vi "Wait for Pulse Acquired.vi"(8 "error in (no error)":errorcluster, 11 "Pulse Recorder Actor in":refnum<class "Pulse Recorder Actor.lvclass">) -> (0 "error out":errorcluster, 3 "Pulse Recorder Actor out":refnum<class "Pulse Recorder Actor.lvclass">)   [LabVIEW 2021, in "Pulse Recorder Actor.lvclass"]
uses:
  Pulse Recorder Actor.lvclass
  C:/GitHub/LabActor/Template Module/Template Module.lvclass
  C:/Program Files/National Instruments/LabVIEW 2021/vi.lib/ActorFramework/Actor/Actor.lvclass
  C:/GitHub/LabActor/Worker/Worker Actor/Worker Actor.lvclass
  Template Module/Template Module.lvclass/Template Module.ctl
  <vilib>/ActorFramework/Actor/Actor.lvclass/Actor.ctl
  Publish-Subscribe/Interfaces/Subscriber Messages/Information Msg/Information Msg.lvclass/Information Msg.ctl
  <vilib>/ActorFramework/Message Enqueuer/Message Enqueuer.lvclass/Message Enqueuer.ctl
  Pulse Recorder Actor.lvclass/Pulse Recorder Actor.ctl
  Interfaces/Pulse Recorder Messages/Wait for Pulse Acquired Msg/Wait for Pulse Acquired Msg.lvclass
  C:/Program Files/National Instruments/LabVIEW 2021/vi.lib/ActorFramework/Message/Message.lvclass
  Worker/Worker Actor/Worker Actor.lvclass/Worker Actor.ctl
  Template Module/Read Name.vi
  Worker/Worker Actor/Read Check again delay.vi
  <vilib>/ActorFramework/Message Enqueuer/Enqueue.vi
  <vilib>/ActorFramework/Message Enqueuer/Init from Existing Queue.vi
  Publish-Subscribe/Interfaces/Subscriber Messages/Information Msg/Information Msg.lvclass
  <vilib>/ActorFramework/Message Priority Queue/Priority Enqueue.vi
  Publish-Subscribe/Interfaces/Information/Information.lvclass
  <vilib>/ActorFramework/Message Enqueuer/Message Enqueuer.lvclass
  <vilib>/ActorFramework/Actor/Actor.lvclass
  C:/GitHub/LabActor/Instrument Actor/Instrument Actor.lvclass
  C:/GitHub/LabActor/Worker/Woker Interface/Worker.lvclass
  C:/GitHub/LabActor/Pulse Recorders/Pulse Recorder Actor/Pulse Recorder Actor.lvclass
  C:/GitHub/LabActor/Pulse Recorders/Interfaces/Pulse Recorder/Pulse Recorder.lvclass
  C:/GitHub/LabActor/Pulse Recorders/Interfaces/Pulse Recorder Messages/Wait for Pulse Acquired Msg/Wait for Pulse Acquired Msg.lvclass
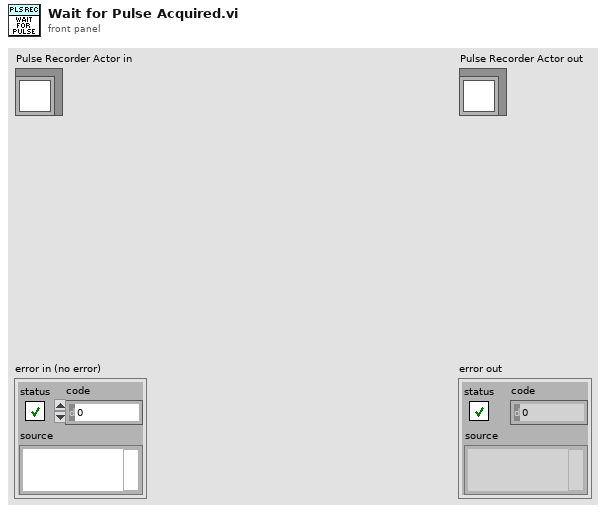
[diagram p1: front panel]
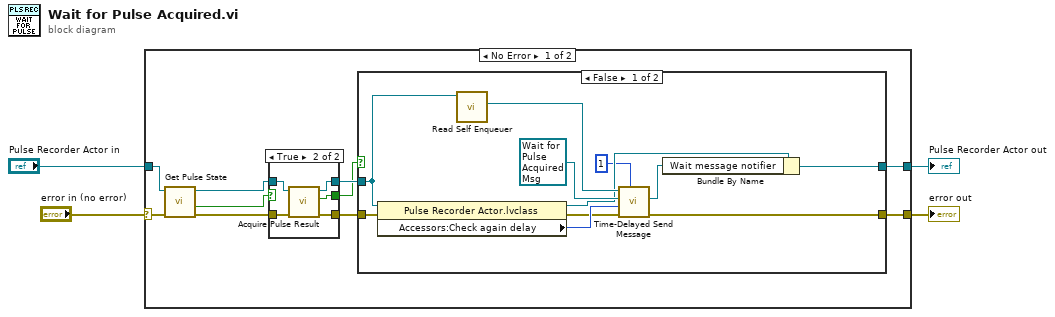
[diagram p0: block diagram]
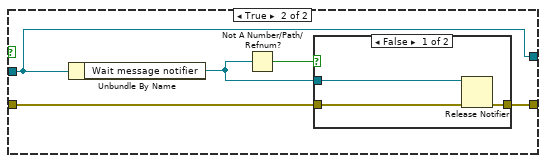
[diagram p2: hidden frame]
diagram:
  n1 = case shown="No Error" "error in (no error)" {
    selector: "error in (no error)" -> [w13 w43]
    tunnel: "Pulse Recorder Actor in" -> [w14 w44]
    tunnel: [w7 w44] -> w2
    tunnel: [w6 w43] -> w1
    frame No Error {
      n2 = call-dynamic "Get Pulse State.vi"("error in (no error)"=w13, "Pulse Recorder Actor in"=w14) -> ("error out"=w11:errorcluster, "Result ready"=w12:bool, "Pulse Recorder Actor out"=w10:refnum<class "Pulse Recorder Actor.lvclass">)  [unwired: 6 in, 1 out]
      n3 = case shown="True" w12 {
        selector: w12 -> [w35 _]
        tunnel: w11 -> [w36 w42]
        tunnel: w10 -> [w37 w41]
        tunnel: [w36 w38] -> w8
        tunnel: [w37 w39] -> w9
        tunnel: [w35 w40] -> w5
        frame False {
        }
        frame True {
          n4 = call-dynamic "Acquire Pulse Result.vi"("error in (no error)"=w42, "Pulse Recorder Actor in"=w41) -> ("error out"=w38:errorcluster, "Pulse acquired"=w40:bool, "Pulse Recorder Actor out"=w39:refnum<class "Pulse Recorder Actor.lvclass">)  [unwired: 7 in]
        }
      }
      n5 = case shown="False" w5 {
        tunnel: w9 -> [w24 w30]
        tunnel: w8 -> [w21 w28]
        tunnel: [w16 w30] -> w7
        tunnel: [w18 w27] -> w6
        frame False {
          n6 = property class="Pulse Recorder Actor.lvclass"(reference=w24, error in=w21) -> (reference out=w20:refnum<class "Pulse Recorder Actor.lvclass">, error out=w19:errorcluster, "Accessors:Check again delay"=w23:i32)
          n7 = call <vilib>:"Read Self Enqueuer.vi"("Actor"=w24) -> ("Self Enqueuer"=w25:refnum<class "Message Enqueuer.lvclass">)  [unwired: 10 in]
          n8 = call <vilib>:"Time-Delayed Send Message.vi"("# Copies (0 = infinite repeat)"=u32 1, "error in (no error)"=w19, "Milliseconds To Wait"=w23, "Message"=refnum<class "Wait for Pulse Acquired Msg.lvclass"> refnum ("Wait for Pulse Acquired Msg.lvclass"), "Message Enqueuer"=w25) -> ("error out"=w18:errorcluster, "Delivery Notifier"=w15:refnum<notifier>)  [unwired: 5 in]
          n9 = Bundle By Name(cluster=w20, "Wait message notifier"=w15) -> (w16:refnum<class "Pulse Recorder Actor.lvclass">)
        }
        frame True {
          n10 = Unbundle By Name(w30) -> ("Wait message notifier"=w26:refnum<notifier>)
          n11 = Not A Number/Path/Refnum?(number/path/refnum=w26) -> (NaN/Path/Refnum?=w29:bool)
          n12 = case shown="False" w29 {
            tunnel: w28 -> [w33 w34]
            tunnel: [w32 w34] -> w27
            tunnel: w26 -> [w31 _]
            frame False {
              n13 = Release Notifier(notifier=w31, error in (no error)=w33) -> (error out=w32:errorcluster)  [unwired: 1 in, 2 out]
            }
            frame True {
            }
          }
        }
      }
    }
    frame Error {
    }
  }
  "error out" <- w1
  "Pulse Recorder Actor out" <- w2
